vi "Inv_Mpemba1_flat potential_withCali.vi"() -> ()   [LabVIEW 2019]
uses:
  <vilib>/eio/EIONode/EIONode.xnode
  <vilib>/rvi/eio/common/nirviEmuTemplateMethod_errors.vi
  <vilib>/eio/EIOPropertyNode/EIOPropertyNode.xnode
  <vilib>/rvi/eio/common/nirviEmuTemplatePropertyGet_errors.vi
  <vilib>/rvi/eio/common/nirviEmuTemplatePropertyGet_noerrors.vi
  <vilib>/rvi/eio/common/nirviEmuTemplatePropertySet_errors.vi
  <vilib>/rvi/eio/common/nirviEmuTemplatePropertySet_noerrors.vi
  <vilib>/rvi/DataTransferAndStorage/Container/XNode/niFpgaContainer.xnode
  <vilib>/rvi/FIFO/Fifo_Resource/nirvififoEmulationWrite.vi
  <vilib>/rvi/FIFO/Fifo_Resource/nirvififoEmulationRead.vi
  <vilib>/rvi/interface/RandomDataEmulation/nirviRandomDataFpgaReadWriteTemplate.vi
panel:
  in  "Bias":sgl
  in  "V_offset":sgl
  in  "Calibration":T1
  in  "Xmin":sgl=-1.0
  in  "Fmax":sgl
  out "num of cycles":sgl
  out "Fx out":sgl
  in  "Xmax":sgl=50.0
  in  "Enum":enum8{"No FB", "HW", "FB"}(ring)
  in  "MobX(px/V)":sgl
  in  "1/Xcali":sgl
  in  "Feedback parameters":T2
  in  "DX":sgl
  in  "DW":cluster{"xm":sgl, "Eb":sgl, "Tau":sgl, "dE":sgl}={"xm"=0.0, "Eb"=0.0, "Tau"=50.0, "dE"=0.0}
  in  "Xmean":sgl
  in  "Calibration ON/OFF":bool
  in  "Frequency":u32=100000
  in  "wait time":sgl=35.0
  in  "Triangle wave":T3={"signal offset_X"=5.0, "Scale X"=0.0, "signal offset_Y"=5.0, "Scale Y"=0.0, "Phase Shift"=30}
  in  "Xoffset":sgl
  in  "Yoffset":sgl
  in  "sum_offset":sgl
  in  "Normalize signal":bool=TRUE
  in  "FB Time":u8=5 caption="Feedback loop time"
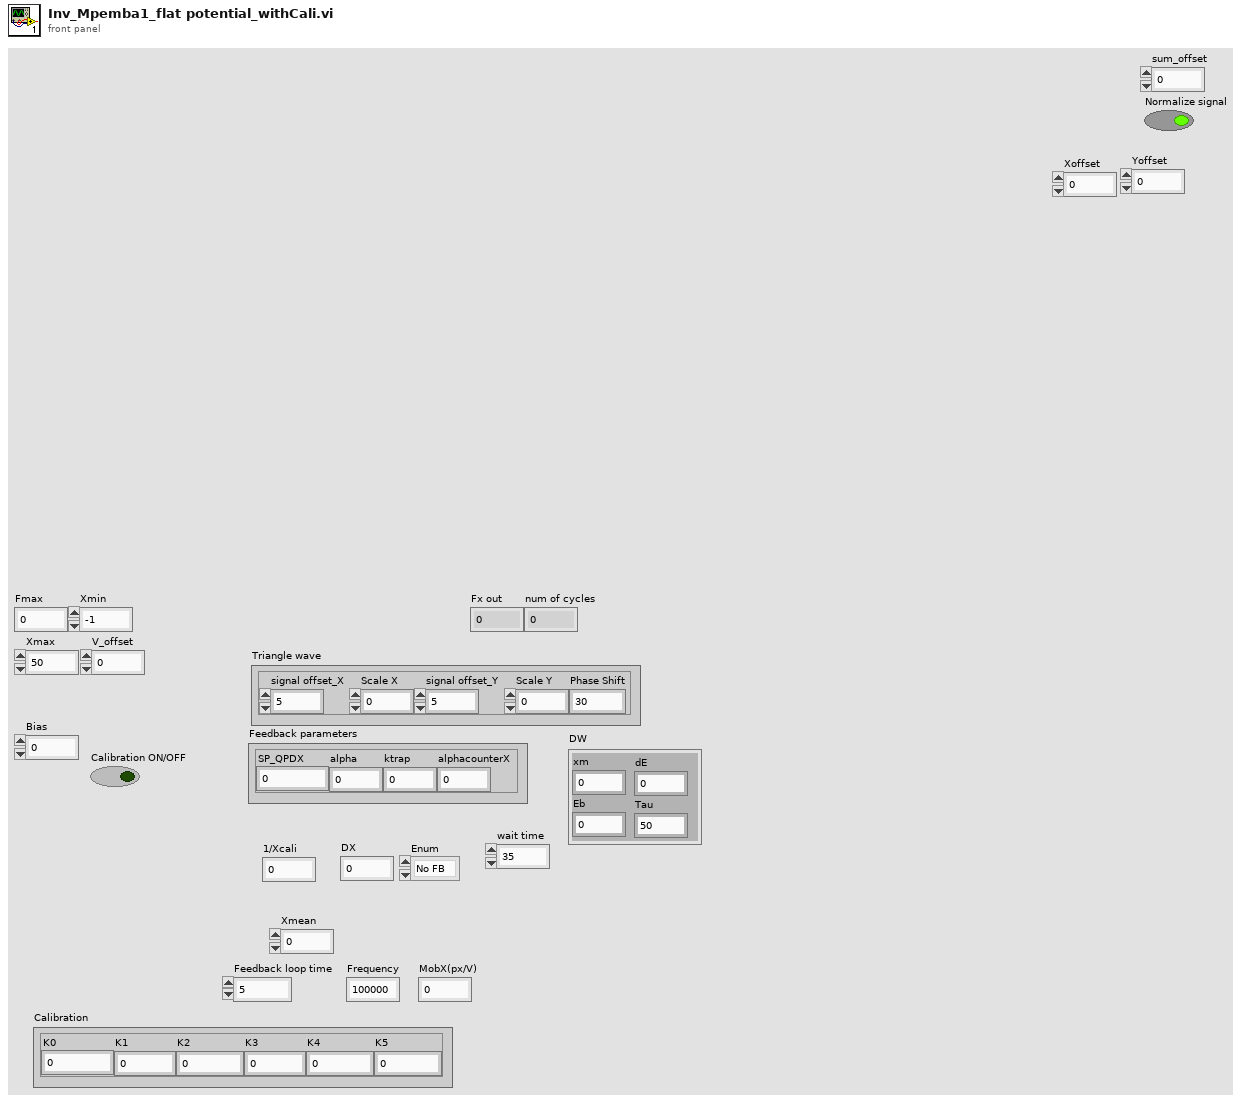
[diagram p1: front panel]
types:
  T1 = cluster{"K0":sgl, "K1":sgl, "K2":sgl, "K3":sgl, "K4":sgl, "K5":sgl}
  T2 = cluster{"SP_QPDX":sgl, "alpha":sgl, "ktrap":sgl, "alphacounterX":sgl}
  T3 = cluster{"signal offset_X":sgl, "Scale X":sgl, "signal offset_Y":sgl, "Scale Y":sgl, "Phase Shift":u32}
  T4 = enum8{"+/- 10 V", "+/- 5 V", "+/- 2 V", "+/- 1 V"}
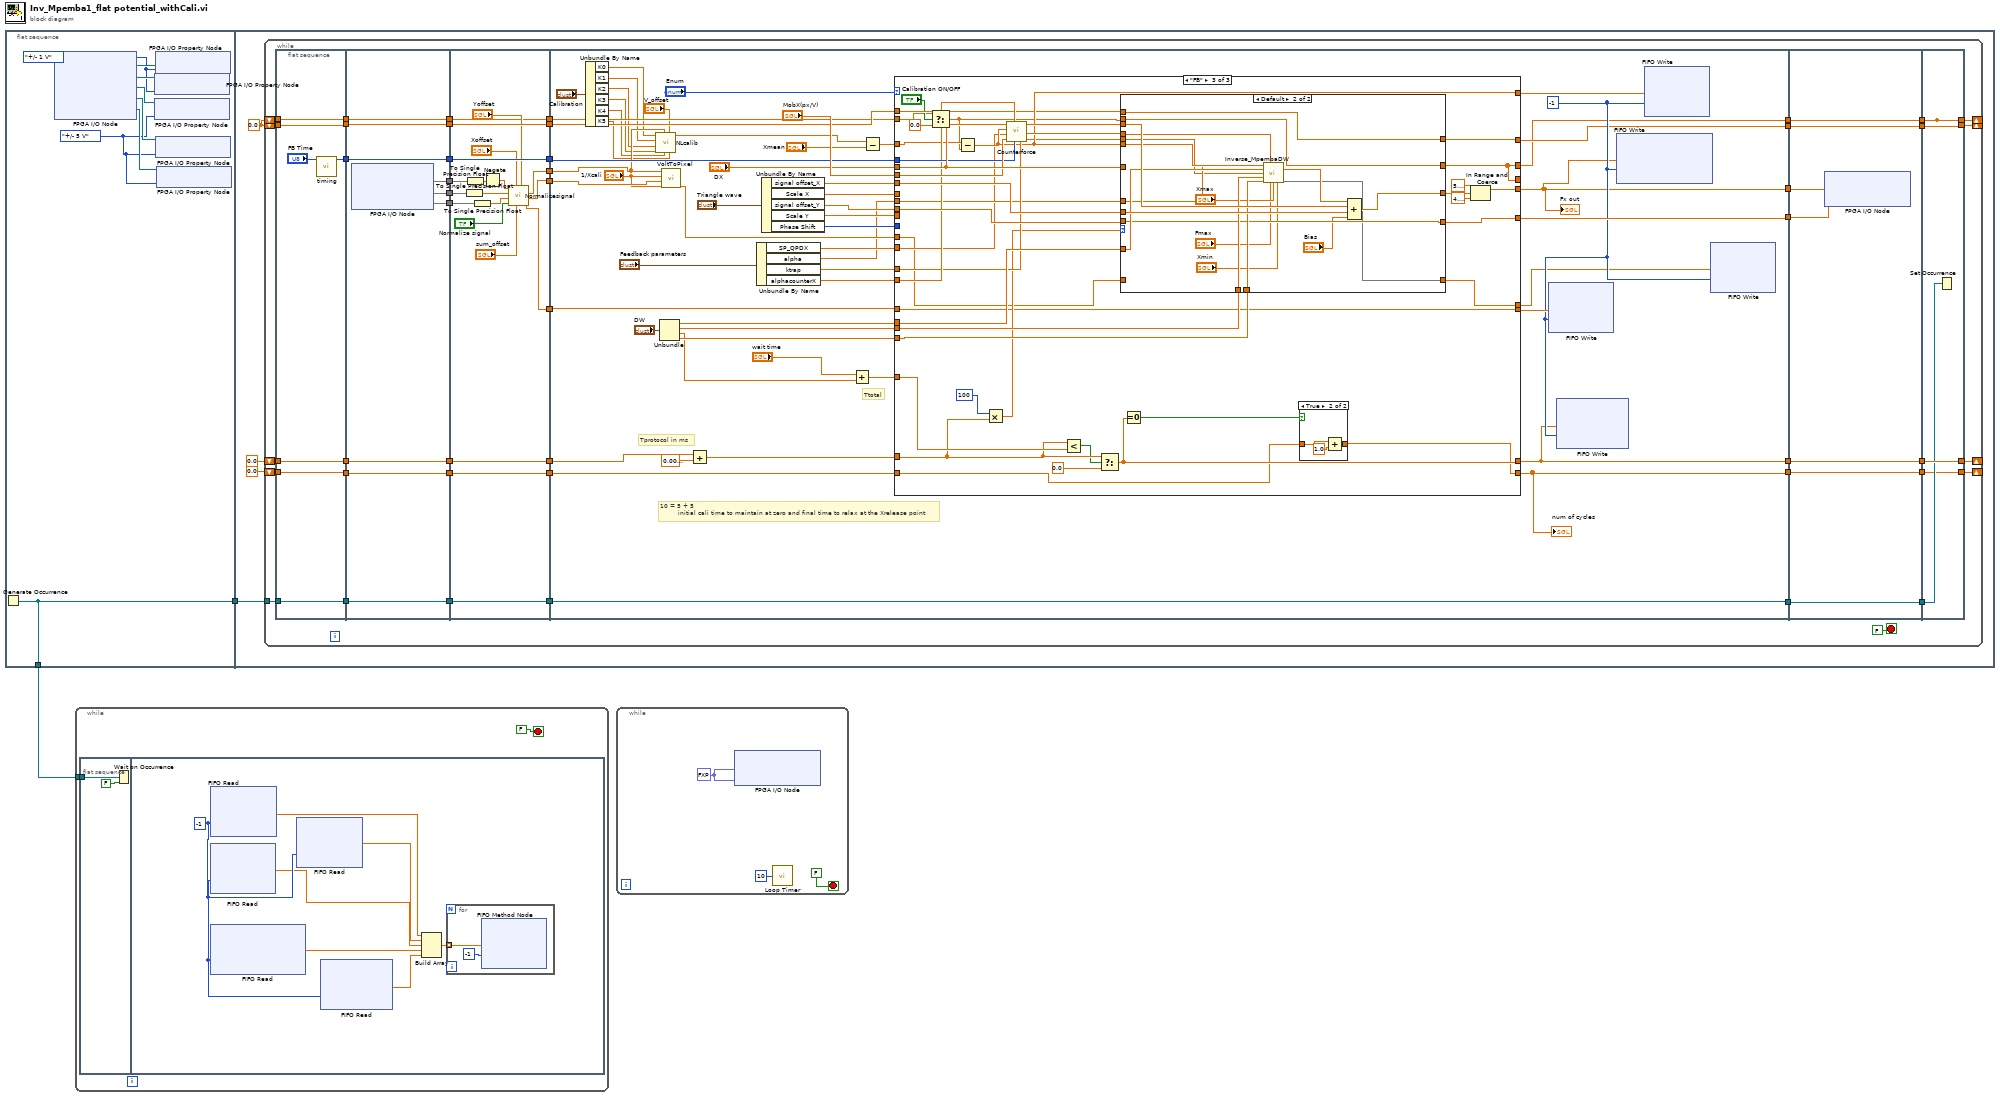
[diagram p0: block diagram]
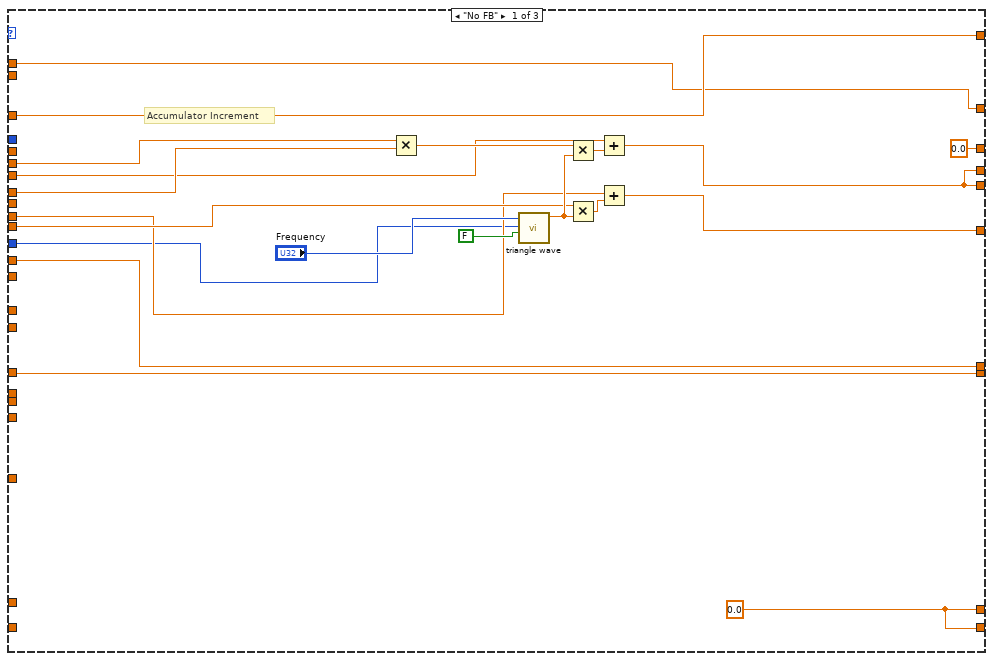
[diagram p2: hidden frame]
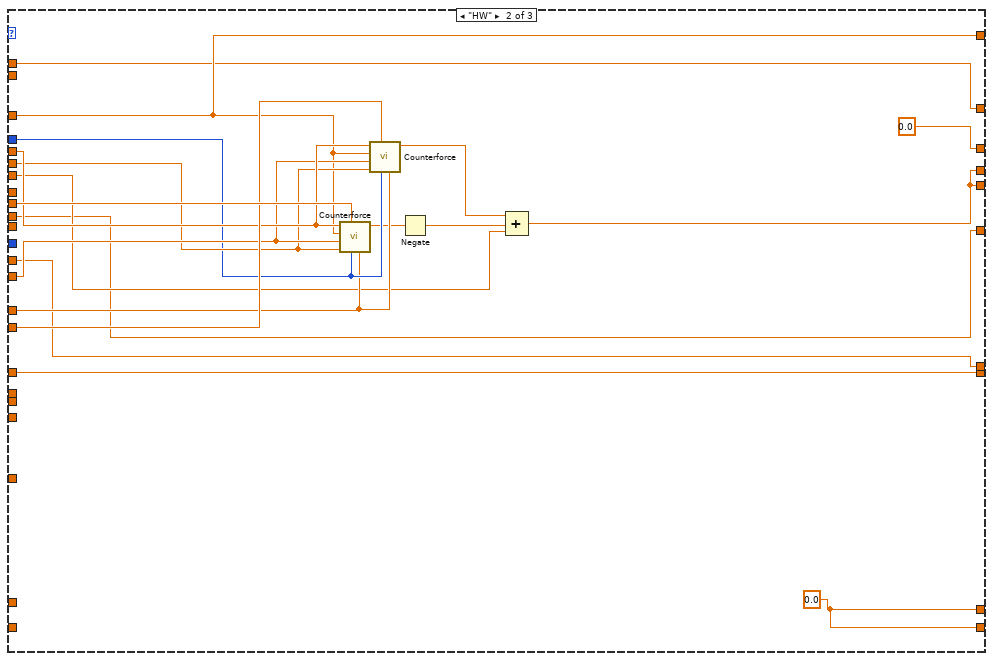
[diagram p3: hidden frame]
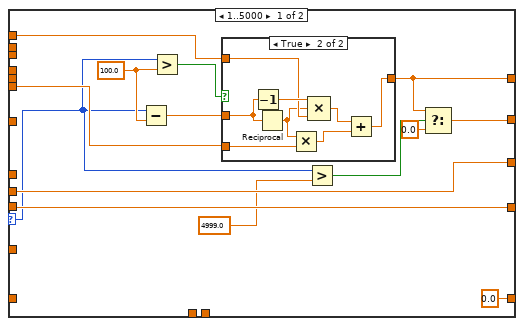
[diagram p4: hidden frame]
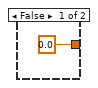
[diagram p5: hidden frame]
diagram:
  n1 = flat-sequence {
    tunnel: [w3] -> w1
    tunnel: [w3] -> w2
    tunnel: w1 -> [w14]
    frame #0 {
      w4 = T4."+/- 5 V" ("Voltage Range")
      w7 = T4."+/- 1 V" ("Voltage Range")
      n2 = Generate Occurrence() -> (w3:refnum<k4>)
      n3 = xnode "FPGA I/O Node"() -> ("FPGA I/O Out"=w10:refnum<k21>, "FPGA I/O Out"=w8:refnum<k21>, "FPGA I/O Out"=w9:refnum<k21>, "FPGA I/O Out"=w5:refnum<k21>, "FPGA I/O Out"=w6:refnum<k21>)  [unwired: 5 in, 5 out]
      n4 = xnode "FPGA I/O Property Node"("FPGA I/O In"=w8, "Voltage Range"=w7) -> ()  [unwired: 1 out]
      n5 = xnode "FPGA I/O Property Node"("FPGA I/O In"=w9, "Voltage Range"=w4) -> ()  [unwired: 1 out]
      n6 = xnode "FPGA I/O Property Node"("FPGA I/O In"=w10, "Voltage Range"=w7) -> ()  [unwired: 1 out]
      n7 = xnode "FPGA I/O Property Node"("FPGA I/O In"=w5, "Voltage Range"=w4) -> ()  [unwired: 1 out]
      n8 = xnode "FPGA I/O Property Node"("FPGA I/O In"=w6, "Voltage Range"=w4) -> ()  [unwired: 1 out]
    }
    frame #1 {
      w11 = sgl 0.0
      n9 = while {
        tunnel: w14 -> [w41]
        shift-right: [w46] -> _
        shift-left: sgl 0.0 -> [w45]
        shift-right: [w33] -> _
        shift-left: w11 -> [w31]
        shift-right: [w26] -> _
        shift-left: sgl 0.0 ("f") -> [w24]
        shift-right: [w19] -> _
        shift-left: w11 -> [w18]
        stop <- FALSE ("stop") stop-if-true
        n10 = flat-sequence {
          tunnel: [w66] -> w49
          tunnel: w45 -> [w65]
          tunnel: [w65] -> w44
          tunnel: w41 -> [w64]
          tunnel: [w64] -> w40
          tunnel: [w63] -> w32
          tunnel: w31 -> [w63]
          tunnel: [w62] -> w25
          tunnel: w24 -> [w62]
          tunnel: w18 -> [w61]
          tunnel: [w61] -> w17
          tunnel: [w76] -> w59
          tunnel: [w75] -> w57
          tunnel: [w74] -> w55
          tunnel: [w73] -> w50
          tunnel: w49 -> [w73]
          tunnel: w44 -> [w72]
          tunnel: [w72] -> w43
          tunnel: w40 -> [w71]
          tunnel: [w71] -> w39
          tunnel: w32 -> [w70]
          tunnel: [w70] -> w29
          tunnel: w25 -> [w69]
          tunnel: [w69] -> w23
          tunnel: w17 -> [w68]
          tunnel: [w68] -> w16
          tunnel: w59 -> [w84]
          tunnel: [w95] -> w58
          tunnel: w57 -> [w83]
          tunnel: [w94] -> w56
          tunnel: w55 -> [w81]
          tunnel: [w93] -> w54
          tunnel: [w96] -> w51
          tunnel: w50 -> [w96]
          tunnel: w43 -> [w92]
          tunnel: [w92] -> w42
          tunnel: w39 -> [w91]
          tunnel: [w91] -> w38
          tunnel: [w89] -> w30
          tunnel: w29 -> [w89]
          tunnel: w23 -> [w88]
          tunnel: [w88] -> w22
          tunnel: w16 -> [w79]
          tunnel: [w79] -> w15
          tunnel: w58 -> [w107]
          tunnel: w56 -> [w147]
          tunnel: w54 -> [w142]
          tunnel: [w97] -> w53
          tunnel: [w151] -> w52
          tunnel: w51 -> [w148]
          tunnel: [w125] -> w48
          tunnel: w42 -> [w144]
          tunnel: w38 -> [w135]
          tunnel: [w135] -> w36
          tunnel: [w127] -> w35
          tunnel: w30 -> [w126]
          tunnel: [w108] -> w28
          tunnel: w22 -> [w124]
          tunnel: [w110] -> w21
          tunnel: w15 -> [w109]
          tunnel: w52 -> [w284]
          tunnel: w53 -> [w285]
          tunnel: w48 -> [w283]
          tunnel: [w283] -> w47
          tunnel: [w282] -> w37
          tunnel: w36 -> [w282]
          tunnel: w35 -> [w281]
          tunnel: [w281] -> w34
          tunnel: w28 -> [w280]
          tunnel: [w280] -> w27
          tunnel: w21 -> [w279]
          tunnel: [w279] -> w20
          tunnel: w47 -> [w290]
          tunnel: [w290] -> w46
          tunnel: w37 -> [w289]
          tunnel: [w288] -> w33
          tunnel: w34 -> [w288]
          tunnel: w27 -> [w287]
          tunnel: [w287] -> w26
          tunnel: w20 -> [w286]
          tunnel: [w286] -> _
          tunnel: [w286] -> w19
          frame #0 {
            n11 = call "timing.vi"("Feedback loop time"="FB Time") -> ("Feedback Loop time"=w66:u32)  [unwired: 10 in]
          }
          frame #1 {
            n12 = xnode "FPGA I/O Node"() -> ("Connector1/AI2"=w76, "Connector1/AI4"=w75, "Connector1/AI5"=w74)  [unwired: 3 in, 3 out]
          }
          frame #2 {
            n13 = To Single Precision Float(number=w83) -> (single precision float=w82:sgl)
            n14 = To Single Precision Float(number=w84) -> (single precision float=w78:sgl)
            n15 = To Single Precision Float(number=w81) -> (single precision float=w80:sgl)
            n16 = Negate(x=w78) -> (-x=w77:sgl)
            n17 = call "Normalizesignal.vi"("Yoffset"="Yoffset", "sum_offset"="sum_offset", "Xoffset"="Xoffset", "Normalize signal"="Normalize signal", "Sum"=w80, "Y"=w82, "X"=w77) -> ("Sum"=w93:sgl, "Y"=w94:sgl, "X"=w95:sgl)  [unwired: 2 in]
          }
          frame #3 {
            w128 = -1 ("Timeout")
            # "10 = 5 + 5\n         initial cali time to maintain at zero and final time to relax at the Xrelease point"
            # "Tprotocol in ms"
            # "Ttotal"
            n18 = Unbundle By Name("Calibration") -> ("K0"=w104:sgl, "K1"=w103:sgl, "K2"=w102:sgl, "K3"=w101:sgl, "K4"=w100:sgl, "K5"=w99:sgl)
            n19 = call "NLcalib.vi"("K5"=w99, "V_offset"="V_offset", "K4"=w100, "Volt QPD"=w107, "K3"=w101, "K2"=w102, "K1"=w103, "K0"=w104) -> ("pixels"=w106:sgl)  [unwired: 3 in]
            n20 = Unbundle("DW") -> ("xm"=w131:sgl, "Eb"=w143:sgl, "Tau"=w112:sgl, "dE"=w137:sgl)
            n21 = call "VoltToPixel.vi"("1/(QPDY/px)"="1/Xcali", "Normalized Y"=w147, "1/(QPDX/px)"="1/Xcali", "Normalized X"=w107) -> ("Ypx"=w146:sgl)  [unwired: 6 in, 1 out]
            n22 = Add(x=w144, y=sgl 0.01) -> (x+y=w136:sgl)
            n23 = Unbundle By Name("Feedback parameters") -> ("SP_QPDX"=w116:sgl, "alpha"=w113:sgl, "ktrap"=w114:sgl, "alphacounterX"=w115:sgl)
            n24 = Unbundle By Name("Triangle wave") -> ("signal offset_X"=w120:sgl, "Scale X"=w122:sgl, "signal offset_Y"=w119:sgl, "Scale Y"=w121:sgl, "Phase Shift"=w118:u32)
            n25 = Add(x="wait time", y=w112) -> (x+y=w145:sgl)
            n26 = Subtract(x=w106, y="Xmean") -> (x-y=w140:sgl)
            n27 = case shown="\"FB\"" "Enum" {
              tunnel: w140 -> [w169 w179 w206]
              tunnel: [w152 w173 w195] -> w97
              tunnel: [w163 w172 w209] -> w151
              tunnel: [w169 w179 w205] -> w139
              tunnel: [w171 w176 w200] -> w138
              tunnel: w142 -> [w171 w176 w200]
              tunnel: w146 -> [w170 w175 w192]
              tunnel: [w170 w175 w191] -> w111
              tunnel: "MobX(px/V)" -> [w162 w186 w229]
              tunnel: w148 -> [_ w185 w220]
              tunnel: "DX" -> [_ w188 w230]
              tunnel: w131 -> [_ _ w227]
              tunnel: w143 -> [_ _ w231]
              tunnel: w136 -> [_ _ w211]
              tunnel: w145 -> [_ _ w222]
              tunnel: [w154 w177 w226] -> w125
              tunnel: w137 -> [_ _ w228]
              tunnel: [w161 w178 w198] -> w127
              tunnel: w126 -> [w161 w178 w203]
              tunnel: [w154 w177 w219] -> w108
              tunnel: w124 -> [_ _ w218]
              tunnel: w122 -> [w159 _ _]
              tunnel: w121 -> [w158 _ _]
              tunnel: w120 -> [w157 w180 w217]
              tunnel: w119 -> [w156 w172 w216]
              tunnel: w118 -> [w155 _ _]
              tunnel: w116 -> [_ w187 w204]
              tunnel: w115 -> [_ w189 w215]
              tunnel: w114 -> [_ w184 w214]
              tunnel: w113 -> [_ w190 w213]
              tunnel: [sgl 0.0 ("f") sgl 0.0 ("f") w194] -> w110
              tunnel: w109 -> [_ _ w196]
              tunnel: [w152 w173 w194] -> _
              frame "No FB" {
                w154 = sgl 0.0 ("f")
                # "Accumulator Increment"
                n28 = Multiply(x=w162, y=w159) -> (x*y=w167:sgl)
                n29 = call "triangle wave.vi"("Reset Accumulator_TW"=FALSE, "phase shift"=w155, "Frequency"="Frequency") -> ("Tri wave out"=w164:sgl)  [unwired: 8 in]
                n30 = Multiply(x=w167, y=w164) -> (x*y=w166:sgl)
                n31 = Multiply(x=w158, y=w164) -> (x*y=w168:sgl)
                n32 = Add(x=w157, y=w166) -> (x+y=w152:sgl)
                n33 = Add(x=w156, y=w168) -> (x+y=w163:sgl)
              }
              frame "HW" {
                w177 = sgl 0.0 ("f")
                n34 = call "Counterforce.vi"("ktrap"=w184, "Ts"=w185, "alphacounterX"=w190, "mobX(px/V)"=w186, "SP_X"=w187, "Xpx"=w179, "Dx"=w188) -> ("counter Force"=w183:sgl)  [unwired: 2 in, 2 out]
                n35 = call "Counterforce.vi"("ktrap"=w184, "Ts"=w185, "alphacounterX"=w189, "mobX(px/V)"=w186, "SP_X"=w187, "Xpx"=w179, "Dx"=w188) -> ("counter Force"=w181:sgl)  [unwired: 2 in, 2 out]
                n36 = Negate(x=w183) -> (-x=w182:sgl)
                n37 = Compound Arithmetic op=ADD(w181, w182, w180) -> (w173:sgl)
              }
              frame "FB" {
                n38 = Select(t=w196, s="Calibration ON/OFF", f=sgl 0.0) -> (s? t:f=w197:sgl)
                n39 = Subtract(x=w206, y=w197) -> (x-y=w205:sgl)
                n40 = Multiply(x=i16 100, y=w211) -> (x*y=w210:sgl)
                n41 = call "Counterforce.vi"("ktrap"=w214, "Ts"=w220, "alphacounterX"=w215, "mobX(px/V)"=w229, "SP_X"=w204, "Xpx"=w205, "Dx"=w230) -> ("Dts"=w193:sgl, "ktrap*mob"=w224:sgl, "counter Force"=w225:sgl)  [unwired: 2 in]
                n42 = Less?(x=w211, y=w222) -> (x < y?=w199:bool)
                n43 = Select(t=w211, s=w199, f=sgl 0.0) -> (s? t:f=w226:sgl)
                n44 = case shown="Default" w210 {
                  selector: w210 -> [w239 _]
                  tunnel: w205 -> [w241 w266]
                  tunnel: w230 -> [_ _]
                  tunnel: [w240 w269] -> w212
                  tunnel: [w245 w268] -> w209
                  tunnel: w216 -> [w245 w268]
                  tunnel: w217 -> [w240 w274]
                  tunnel: w213 -> [_ w258]
                  tunnel: w227 -> [_ w272]
                  tunnel: w231 -> [_ w271]
                  tunnel: w225 -> [_ w273]
                  tunnel: w224 -> [_ w263]
                  tunnel: w228 -> [_ w270]
                  tunnel: [w236 w267] -> w198
                  tunnel: w203 -> [w242 w267]
                  tunnel: [w234 w264] -> w194
                  tunnel: w197 -> [_ w264]
                  tunnel: w193 -> [_ w257]
                  tunnel: w192 -> [_ _]
                  tunnel: [sgl 0.0 ("Protocol output") w256] -> w191
                  frame 1..5000 {
                    w246 = sgl 100.0 ("y")
                    n45 = Subtract(x=w239, y=w246) -> (x-y=w243:sgl)
                    n46 = Greater?(x=w239, y=w246) -> (0:w244:bool)
                    n47 = case shown="True" w244 {
                      tunnel: [sgl 0.0 w249] -> w236
                      tunnel: w243 -> [_ w255]
                      tunnel: w242 -> [_ w253]
                      tunnel: w241 -> [_ w252]
                      frame False {
                      }
                      frame True {
                        n48 = Decrement(x=w255) -> (x-1=w254:sgl)
                        n49 = Reciprocal(x=w255) -> (1/x=w248:sgl)
                        n50 = Multiply(x=w248, y=w252) -> (x*y=w250:sgl)
                        n51 = Compound Arithmetic op=MULTIPLY(w254, w248, w253) -> (w251:sgl)
                        n52 = Add(x=w251, y=w250) -> (x+y=w249:sgl)
                      }
                    }
                    n53 = Greater?(x=w239, y=sgl 4999.0) -> (0:w237:bool)
                    n54 = Select(t=w236, s=w237, f=sgl 0.0) -> (s? t:f=w234:sgl)
                  }
                  frame Default {
                    n55 = call "Inverse_MpembaDW.vi"("Xpos"=w266, "ktrap*mob"=w263, 4:w258, "Xm"=w272, 7:w257, "Eb"=w271, "dE"=w270, "Fmax"="Fmax", "Xmax"="Xmax", "Xmin"="Xmin") -> ("DWvolt"=w265:sgl, 15:w256)  [unwired: 4 in]
                    n56 = Compound Arithmetic op=ADD(w265, w273, w274, "Bias") -> (w269:sgl)
                  }
                }
                n57 = Equal To 0?(x=w226) -> (x = 0?=w223:bool)
                n58 = case shown="True" w223 {
                  tunnel: [w275 w278] -> w219
                  tunnel: w218 -> [w275 w277]
                  frame False {
                  }
                  frame True {
                    n59 = Add(x=w277, y=sgl 1.0) -> (x+y=w278:sgl)
                  }
                }
                n60 = In Range and Coerce(upper limit=sgl 5.1, x=w212, lower limit=sgl 4.9) -> (coerced(x)=w195:sgl)  [unwired: 1 out]
              }
            }
            "Fx out" <- w97
            "num of cycles" <- w108
            n61 = xnode ("FIFO Write")("Element"=w138, "Timeout"=w128) -> ()  [unwired: 1 in, 2 out]
            n62 = xnode ("FIFO Write")("Element"=w125, "Timeout"=w128) -> ()  [unwired: 1 in, 2 out]
            n63 = xnode ("FIFO Write")("Element"=w97, "Timeout"=w128) -> ()  [unwired: 1 in, 2 out]
            n64 = xnode ("FIFO Write")("Element"=w139, "Timeout"=w128) -> ()  [unwired: 1 in, 2 out]
            n65 = xnode ("FIFO Write")("Element"=w111, "Timeout"=w128) -> ()  [unwired: 1 in, 2 out]
          }
          frame #4 {
            n66 = xnode "FPGA I/O Node"("Connector1/AO7"=w285, "Connector1/AO6"=w284) -> ()  [unwired: 2 in, 2 out]
          }
          frame #5 {
            n67 = Set Occurrence(w289) -> ()
          }
        }
      }
    }
  }
  n68 = while {
    tunnel: w2 -> [w291]
    stop <- FALSE stop-if-true
    n69 = flat-sequence {
      tunnel: w291 -> [w294]
      frame #0 {
        n70 = Wait on Occurrence(1:FALSE ("ignore previous (T)"), 2:w294) -> ()  [unwired: 1 in, 1 out]
      }
      frame #1 {
        w297 = -1 ("Timeout")
        n71 = xnode ("FIFO Read")("Timeout"=w297) -> ("Element"=w295:sgl)  [unwired: 1 in, 2 out]
        n72 = xnode ("FIFO Read")("Timeout"=w297) -> ("Element"=w298:sgl)  [unwired: 1 in, 2 out]
        n73 = xnode ("FIFO Read")("Timeout"=w297) -> ("Element"=w299:sgl)  [unwired: 1 in, 2 out]
        n74 = xnode ("FIFO Read")("Timeout"=w297) -> ("Element"=w296:sgl)  [unwired: 1 in, 2 out]
        n75 = xnode ("FIFO Read")("Timeout"=w297) -> ("Element"=w300:sgl)  [unwired: 1 in, 2 out]
        n76 = Build Array(w299, w296, w295, w298, w300) -> (w301:sgl[])
        n77 = for {
          tunnel: w301 -> [w303] mode=indexing
          n78 = xnode ("FIFO Method Node")("Element"=w303, "Timeout"=-1) -> ()  [unwired: 1 in, 2 out]
        }
      }
    }
  }
  n79 = while {
    stop <- FALSE stop-if-true
    w304 = fxp<+,8,3> 2.5 ("Connector1/AO2")
    n80 = xnode "FPGA I/O Node"("Connector1/AO0"=w304, "Connector1/AO4"=w304) -> ()  [unwired: 2 in, 2 out]
    n81 = call "Loop Timer"("Count(uSec)"=u8 10) -> ()  [unwired: 1 out]
  }
